vi "Initialize Front Panel.vi"(8 "error in (no error)":errorcluster, 11 "Alpha View in":refnum<class "Alpha View.lvclass">) -> (0 "error out":errorcluster, 3 "Alpha View out":refnum<class "Alpha View.lvclass">)   [LabVIEW 2017, in "Alpha View.lvclass"]
doc: "<License>\nCopyright © 2017 Composed Systems, LLC | All rights reserved\nwww.composed.io\n\nAuthor: Ethan Stern <ethan.stern@composed.io>\n\nThis software is provided \"AS IS\" WITHOUT WARRANTIES, either express or implied, AND IS FOR EDUCATIONAL PURPOSES ONLY.\n</License>"
uses:
  <vilib>/gpm_packages/@cs/popup-viewmanager/Example/Alpha View/Alpha View.lvclass
  <vilib>/gpm_packages/@cs/popup-viewmanager/Example/Alpha View/Alpha View.lvclass/Alpha View.ctl
  <vilib>/gpm_packages/@cs/mva-viewable/Source/IViewable/IViewable/IViewable.lvclass
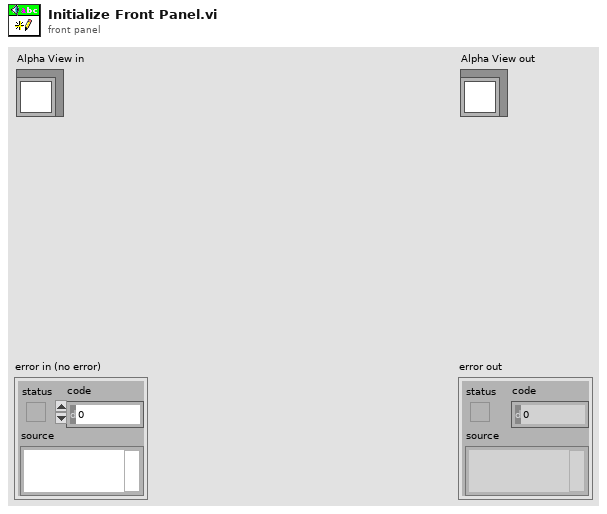
[diagram p1: front panel]
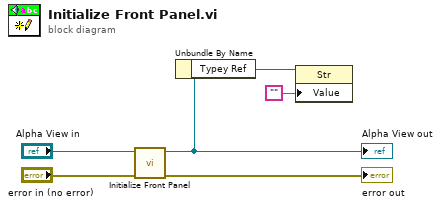
[diagram p0: block diagram]
diagram:
  n1 = call-parent "Initialize Front Panel.vi"("error in (no error)"="error in (no error)", "IViewable in"="Alpha View in") -> ("error out"=→"error out":errorcluster, "IViewable out"=w3:refnum<class "Alpha View.lvclass">)  [unwired: 8 in]
  "Alpha View out" <- w3
  n2 = Unbundle By Name(w3) -> ("Typey Ref"=w2:refnum<vi>)
  n3 = property class="Str"(reference=w2, "Value"="") -> ()  [unwired: 1 in, 2 out]
